vi "play-raster-scan.vi"() -> ()   [LabVIEW 2017]
uses:
  raster-scan-params.ctl
  controls/PI-params.ctl
  controls/boolean_info.ctl
  controls/raster_input_meta_data.ctl
  <vilib>/userdefined/High Color/nirio_resource_hc.ctl
  controls/rasterMetaData.ctl
  <vilib>/Utility/file.llb/Read Delimited Spreadsheet (DBL).vi
  <vilib>/FPGAPlugInAG/cRIO-9082/niLvFpga_Open_cRIO-9082.vi
  <vilib>/rvi/interface/common/dynamic/niFpgaDynamicAddResources.vi
  <vilib>/FPGAPlugInAG/Dynamic/niLvFpga_Reset_Dynamic.vi
  <vilib>/rvi/interface/common/niFpgaWaitOnOcc.vi
  <vilib>/Utility/error.llb/Error Cluster From Error Code.vi
  <vilib>/rvi/errors/niLvFpgaAdjustHostInterfaceError.vi
  <vilib>/FPGAPlugInAG/Dynamic/niLvFpga_Run_Dynamic.vi
  <vilib>/FPGAPlugInAG/Dynamic/niLvFpga_Close_Dynamic.vi
  <userlib>/_matio/level5/Public/Write/Append Data Element.llb/Append Data Element (Anything).vi
  <vilib>/rvi/interface/nirviOpenFPGA/nirviOpenFPGA.xnode
  FPGA Bitfiles/afmimagingcontro_FPGATargetSPARTA_raster-scanning_DXF4O8EAjZ4.lvbitx
  <vilib>/rvi/interface/nirviMethod/nirviMethod.xnode
  <vilib>/rvi/interface/nirviReadWriteControl/nirviReadWriteControl.xnode
  <vilib>/rvi/interface/nirviCloseFPGA/nirviCloseFPGA.xnode
  <vilib>/FPGAPlugInAG/Dynamic/niLvFpga_ConfigureFifo_Dynamic.vi
  <vilib>/rvi/errors/niLvFpgaMergeErrorWithErrorCode.vi
  <vilib>/rvi/interface/Simulation/niFpgaSimulationCallBeginRW.vi
  <vilib>/FPGAPlugInAG/Dynamic/niLvFpga_ReadFifo_Dynamic.vi
  NiFpgaLv.dll
  <userlib>/_matio/level5.lvlib
  <vilib>/FPGAPlugInAG/Dynamic/niLvFpga_WriteFifo_Dynamic.vi
panel:
  in  "detrend":bool=TRUE
  out "control":dbl[](graph)
  out "error":dbl[](graph)
  out "InputMetaData":T1
  out "output-meta-data-path":path
  in  "Tab Control":enum32{"Page 1", "Debug"}(tab)
  in  "data-root":path=path "C:/Users/arnold/Documents/labview/afm_imaging/data/raster/5microns"
  in  "number-of-pixels":i32=512
  out "points_per_line":i32=250000
  out "total_num_points":i32
  in  "raise-constant (init)":sgl
  in  "raise-constant":sgl
  in  "trigger-0":bool
  in  "STOP":bool
  in  "xy-init":fxp<+/-,16,5>[](array[numeric])=[0.0, 0.0]
  in  "Ki-xy":dbl=0.01 format="%#_13g"
  out "ADC-zaxis":sgl
  out "DAC-zaxis":sgl
  in  "xy-bound":sgl=7.0
  out "output-data-path":path
  in  "input-data-file-name":string="raster_scan_5mic_1Hz.csv"
  in  "note-blob":string
  in  "overwrite":bool
  in  "raster-scan-params":T2={"TsTicks"=1600, "Stop"=TRUE, "TOL"=0.3, "ramp-rate"=-5e-05, "z-u-max"=5.0, "PI-params"={"Ki"=0.01, "setpoint"=0.0}, "Num"=[1.0, 0.0, 0.0, 0.0, 0.0, 0.0, 0.0, 0.0, 0.0], "TF Order"=1, "Den"=[1.0, 0.0, 0.0, 0.0, 0.0, 0.0, 0.0, 0.0, 0.0]} {"ramp-rate" format="%#_5g"; "TOL" format="%#_13g"}
  in  "do-Dz":bool
  in  "do_xy_CL":bool
  out "boolean errors":T4
  in  "Z-settle-N":i16=10000
  out "Actual Depth":u32
  out "Elements Remaining":u32
  out "size(s)":i32
  out "y iter":i32
  out "nsamps 2":i32
  out "Empty Elements Remaining":u32
  out "(int) y*floor(x/y)":u64
  out "elements left 2":i32=1
  out "x >= y?":bool
  out "writing stopped":bool
  out "size(s) 2":i32
  out "case-selector-feedback":i16
  out "e(0) (threshhold init)":fxp<+/-,16,5>
  out "total-time":dbl
  out "x+1":i32
  out "que timed out?":bool
  out "Error signal (previous line) 2":dbl[](graph)
  out "Waveform Graph":dbl[](graph)
  out "base y_ref (ramp)":dbl[](graph)
  out "base x_ref(triangle wave)":dbl[](graph)
  out "Intensity Graph":dbl[][](graph)
  out "Error signal (previous line)":dbl[](graph)
  # "x-axis"
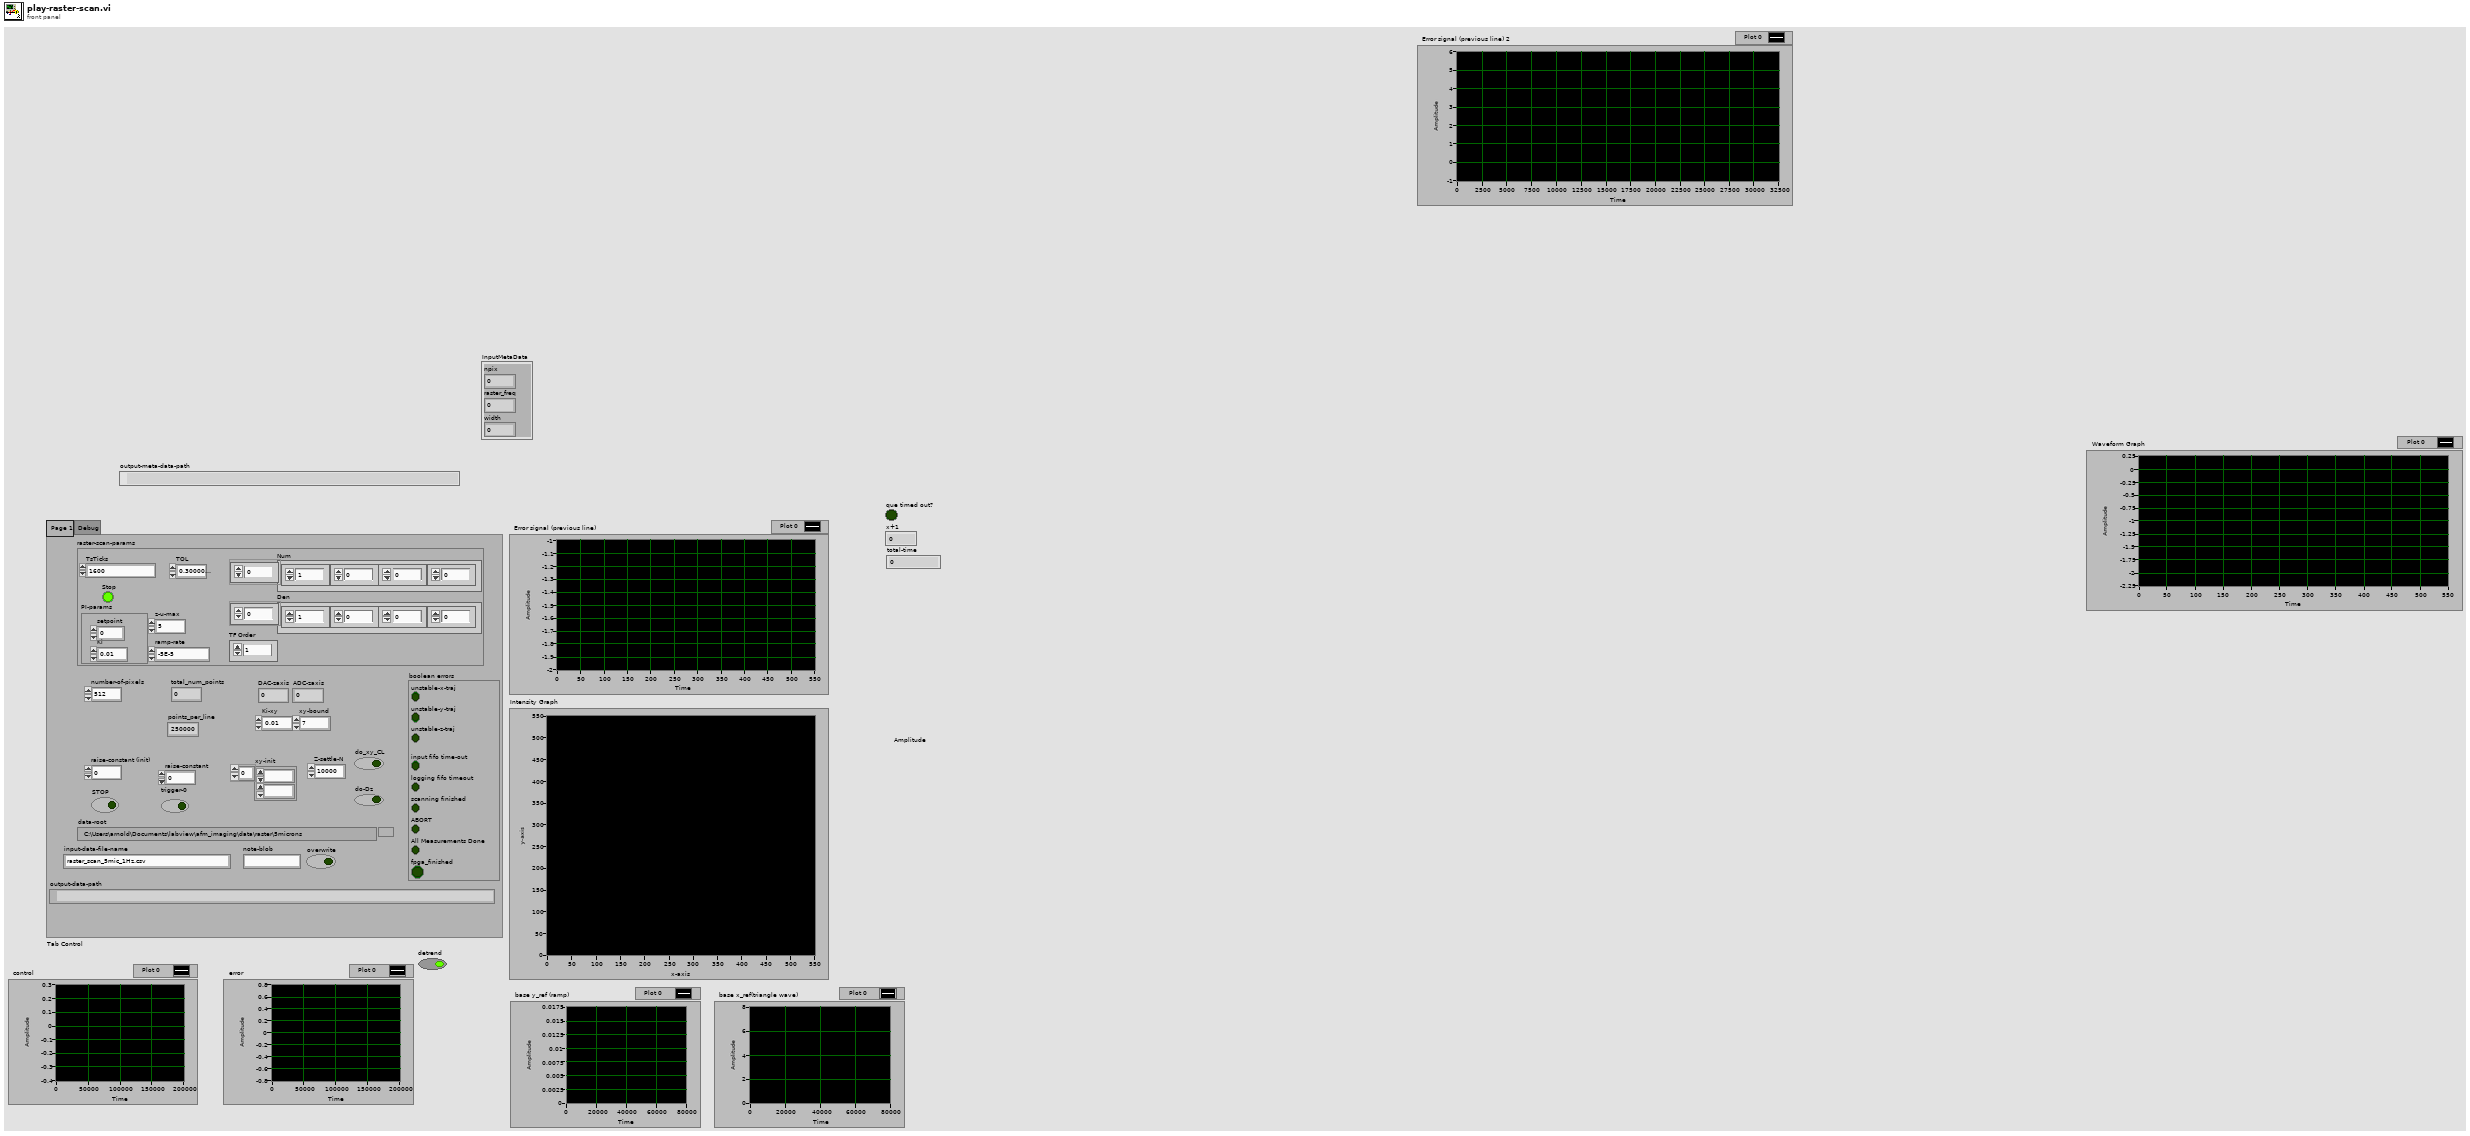
[diagram p1: front panel]
types:
  T1 = typedef "raster_input_meta_data.ctl" = cluster{"npix":dbl, "raster_freq":dbl, "width":dbl}
  T2 = typedef "raster-scan-params.ctl" = cluster{"TsTicks":u32, "Stop":bool, "TOL":sgl, "ramp-rate":sgl, "z-u-max":sgl, "PI-params":T3, "Num":sgl[], "TF Order":i32, "Den":sgl[]}
  T3 = typedef "PI-params.ctl" = cluster{"Ki":sgl, "setpoint":sgl}
  T4 = typedef "boolean_info.ctl" = cluster{"unstable-z-traj":bool, "input fifo time-out":bool, "logging fifo timeout":bool, "scanning finished":bool, "unstable-x-traj":bool, "unstable-y-traj":bool, "ABORT":bool, "All Measurements Done":bool, "fpga_finished":bool}
  T5 = typedef "nirio_resource_hc.ctl" = tag
  T6 = enum16{"open", "replace", "create", "open or create", "replace or create", "replace or create with confirmation"}
  T7 = cluster{"unstable-z-traj":bool, "input fifo time-out":bool, "logging fifo timeout":bool, "scanning finished":bool, "unstable-x-traj":bool, "unstable-y-traj":bool, "ABORT":bool, "All Measurements Done":bool, "fpga_finished":bool}
  T8 = typedef "rasterMetaData.ctl" = cluster{"raster-scan-params":T2, "xy-bound":sgl, "DAC-zaxis":sgl, "ADC-zaxis":sgl, "Ki-xy":dbl, "total_num_points":i32, "points_per_line":i32, "number-of-lines":i32, "number-of-pixels":i32, "raster_meta_in":T1}
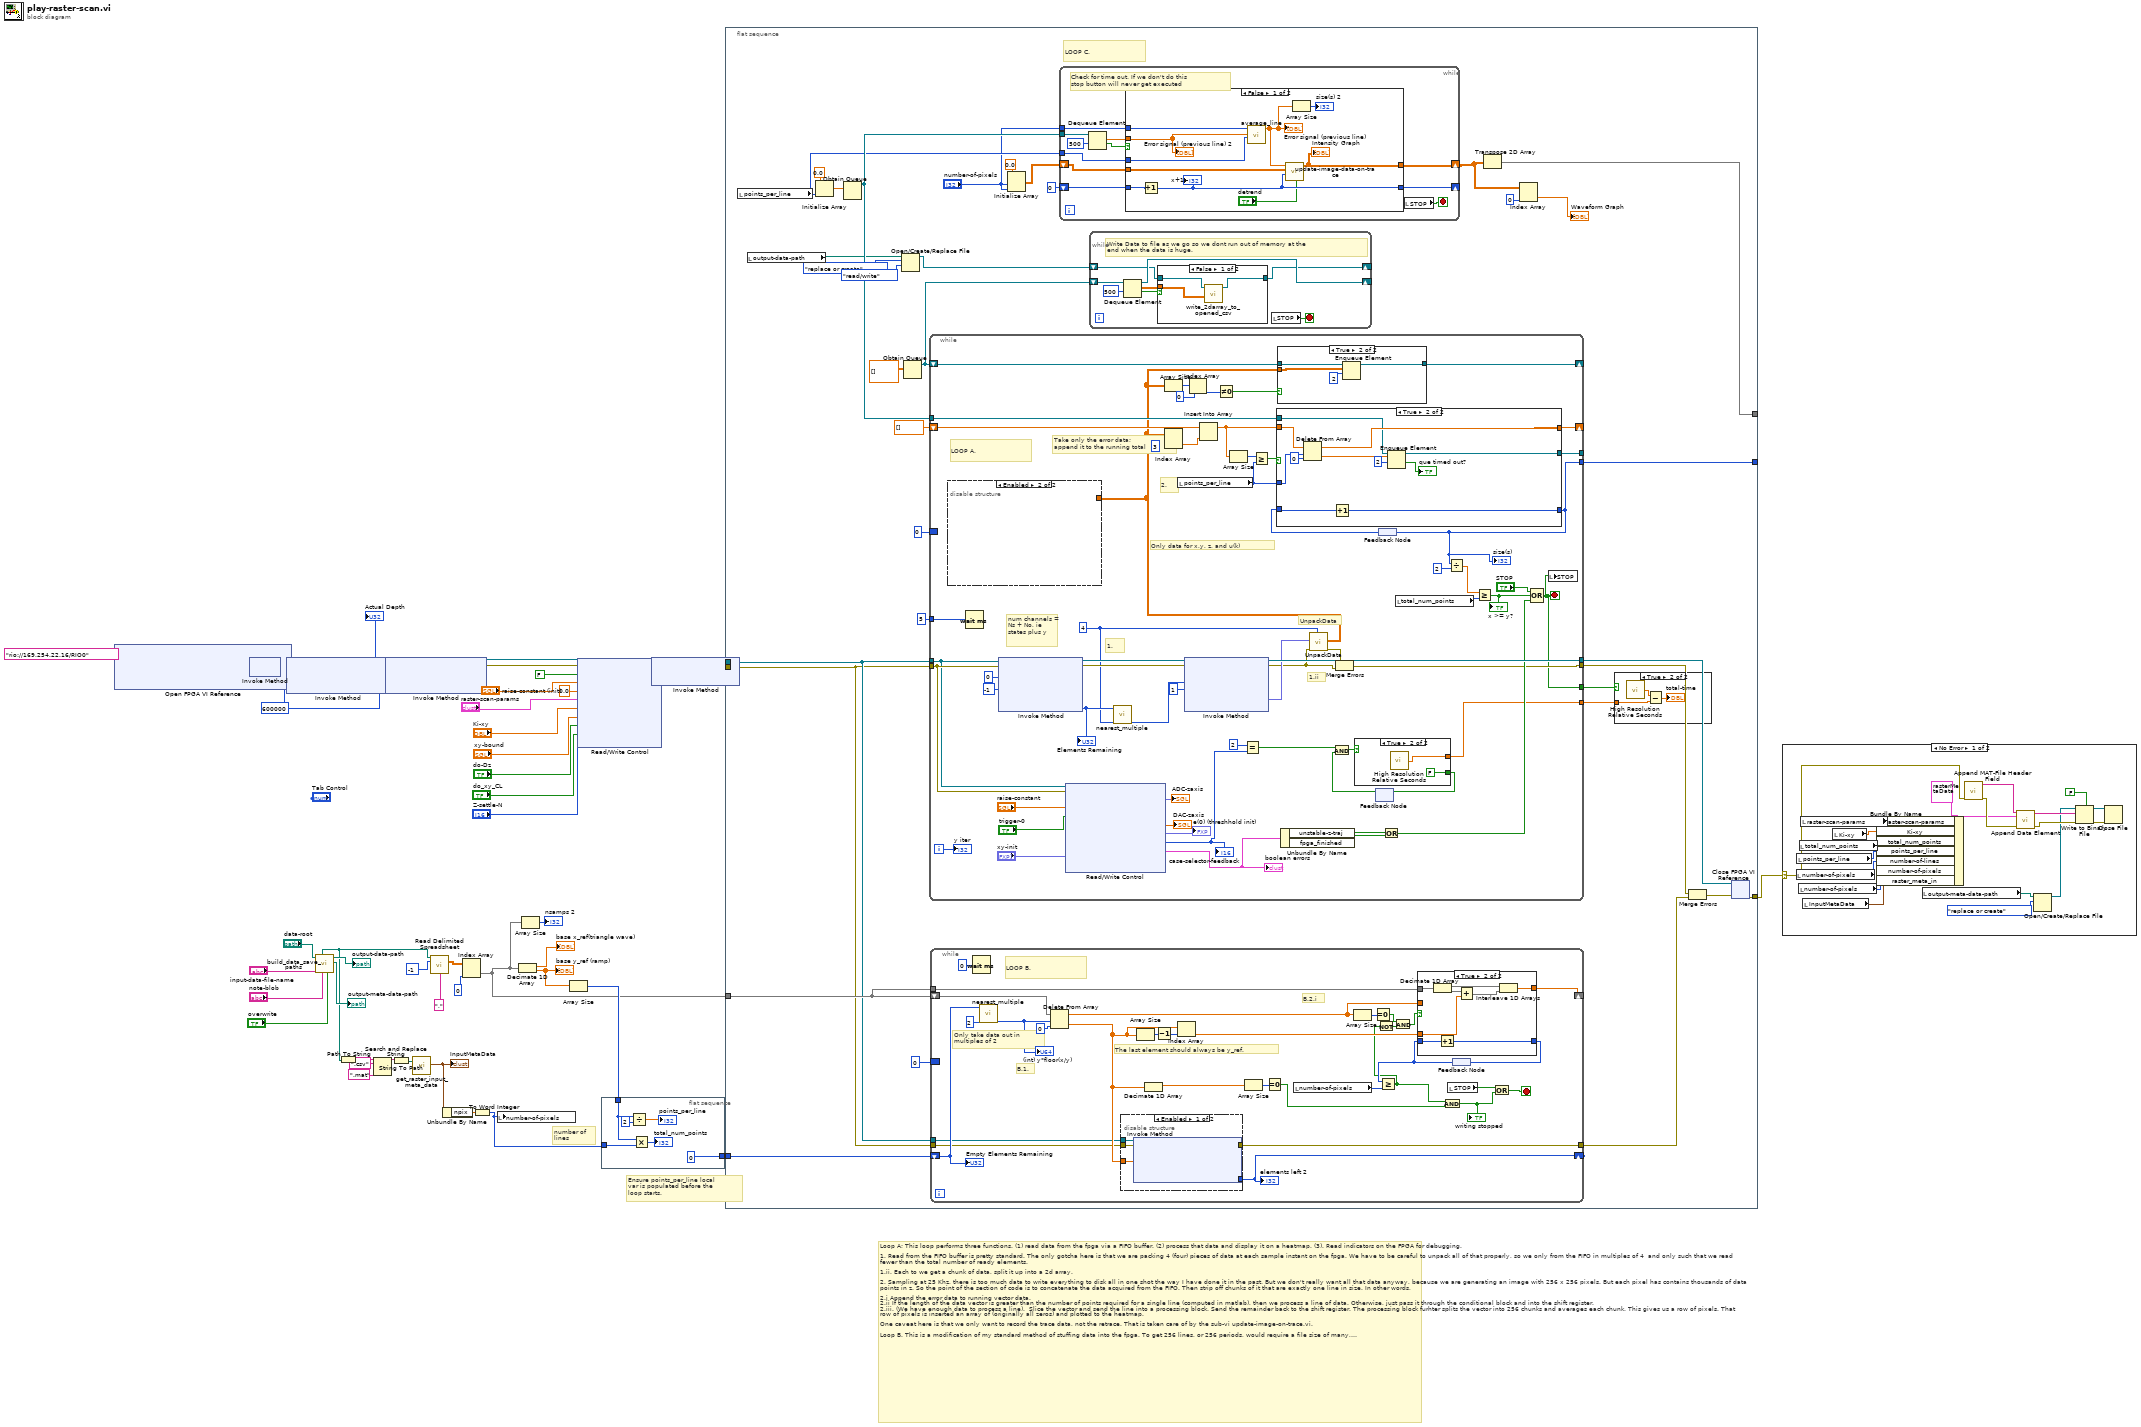
[diagram p0: block diagram]
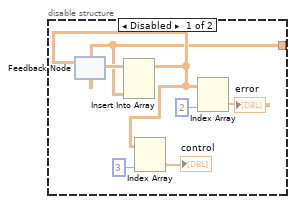
[diagram p6: hidden frame]
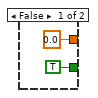
[diagram p8: hidden frame]
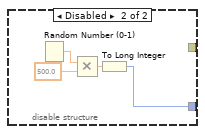
[diagram p11: hidden frame]
diagram:
  w48 = 600000
  # "number of \nlines"
  # "Loop A; This loop performs three functions. (1) read data from the fpga via a FIFO buffer. (2) process that data and display it on a heatmap. (3). Read indicators on the FPGA for debugging.\n\n1. Read from the FIFO buffer is pretty standard. The only gotcha here is that we are packing 4 (four) pieces of data at each sample instant on the fpga. We have to be careful to unpack all of that properly, so we only from the FIFO in multiples of 4  and only such that we read fewer than the total number of ready elements. \n\n1.ii. Each to we get a chunk of data, split it up into a 2d array. \n\n2. Sampling at 25 Khz, there is too much data to write everything to disk all in one shot the way I have done it in the past. But we don't really want all that data anyway, because we are generating an image with 256 x 256 pixels. But each pixel has contains thousands of data points in z. So the point of the section of code is to concatenate the data acquired from the FIFO. Then strip off chunks of it that are exactly one line in size. In other words,\n\n2.i Append the error data to running vector data.\n2.ii If the length of the data vector is greater than the number of points required for a single line (computed in matlab), then we process a line of data. Otherwise, just pass it through the conditional block and into the shift register. \n2.iii. (We have enough data to process a line).  Slice the vector and send the line into a processing block. Send the remainder back to the shift register. The processing block furhter splits the vector into 256 chunks and averages each chunk. This gives us a row of pixels. That row of pixels is inserted an array of (originally all zeros) and plotted to the heatmap.\n\nOne caveat here is that we only want to record the trace data, not the retrace. That is taken care of by the sub-vi update-image-on-trace.vi.\n\nLoop B. This is a modification of my standard method of stuffing data into the fpga. To get 256 lines, or 256 periods, would require a file size of many, many gigibtyes. SO the point here is to only use a single period of the triangle wave and corresponding ramp signal. Everytime we exauhst that data, re-cycle the same data and keep pumping it back in. The one tricky part here is that we have to be careful to shift the original ramp data up by the appropriate amount. We also have to take special care because of how the data is packed from matlab. [x(1), y(1), x(2), y(2)...].\n\nThe first iteration of the loop, we don't push any data in. All we do is get the number of empty elements.\n\nB.1 Each iteration, strip off ' empty elements ' elements from the array and send them to FIFO. \nB.2.i Is the remaining array empty?\nB.2.ii Grab the very last element. We need this"
  # "Ensure points_per_line local\nvar is populated before the\nloop starts."
  n1 = xnode "Open FPGA VI Reference"("resource name"=T5 "rio://169.254.22.16/RIO0") -> ("FPGA VI Reference Out"=w47:refnum<k20>, "error out"=w46:errorcluster)  [unwired: 1 in]
  n2 = xnode "Invoke Method"("FPGA VI Reference In"=w47, "error in"=w46) -> ("FPGA VI Reference Out"=w42:refnum<k20>, "error out"=w41:errorcluster)
  n3 = xnode "Invoke Method"("FPGA VI Reference In"=w42, "error in"=w41, "Requested Depth"=w48) -> ("FPGA VI Reference Out"=w43:refnum<k20>, "error out"=w44:errorcluster, "Actual Depth"=→"Actual Depth":u32)
  n4 = call "build_data_save_paths.vi"("overwrite"="overwrite", "note-blob"="note-blob", "base-file-name"="input-data-file-name", "data-root"="data-root") -> ("output-meta-data-path"=→"output-meta-data-path":path, "output-data-path"=→"output-data-path":path, "input-data-path"=w9:path)  [unwired: 3 in, 2 out]
  n5 = Path To String(path=w9) -> (string=w8:string)
  n6 = Search and Replace String(input string=w8, search string=".csv", replace string=".mat" ("replace string (\"\")")) -> (result string=w5:string)  [unwired: 5 in, 3 out]
  n7 = xnode "Invoke Method"("FPGA VI Reference In"=w43, "error in"=w44, "Requested Depth"=w48) -> ("FPGA VI Reference Out"=w50:refnum<k20>, "error out"=w49:errorcluster)  [unwired: 1 out]
  n8 = String To Path(string=w5) -> (path=w4:path)
  n9 = call "get_raster_input_meta_data.vi"("Path"=w4) -> ("cluster"=w3:T1)  [unwired: 10 in]
  "InputMetaData" <- w3
  n10 = call-poly <vilib>:"Read Delimited Spreadsheet.vi"("file path (dialog if empty)"=w9, "number of rows (all:-1)"=-1, "delimiter (\\t)"=",") -> ("all rows"=w28:dbl[][])  [unwired: 7 in, 5 out]
  n11 = Unbundle By Name(w3) -> ("npix"=w2:dbl)
  n12 = Index Array(array=w28, index (col)=0 ("dimension size")) -> (element=w27:dbl[])  [unwired: 1 in]
  n13 = To Word Integer(number=w2) -> (16bit integer=w1:i16)
  n14 = local write "number-of-pixels"(w1) -> ()
  n15 = Decimate 1D Array(w27) -> (→"base x_ref(triangle wave)":dbl[], w34:dbl[])
  "base y_ref (ramp)" <- w34
  n16 = Array Size(array=w27) -> (size(s)=→"nsamps 2":i32)
  n17 = Array Size(array=w34) -> (size(s)=w32:i32)
  n18 = xnode "Read/Write Control"("FPGA VI Reference In"=w50, "error in"=w49, "trigger-0"=FALSE ("constant 2 lower"), "raise-constant"="raise-constant (init)", "u(0)"=sgl 0.0, "raster-scan-params"="raster-scan-params", "Ki-xy"="Ki-xy", "xy-bound"="xy-bound", "do-Dz"="do-Dz", "do_xy_CL"="do_xy_CL", "Z-settle-N"="Z-settle-N") -> ("FPGA VI Reference Out"=w24:refnum<k20>, "error out"=w23:errorcluster)
  n19 = flat-sequence {
    tunnel: [0] -> w33
    tunnel: w32 -> [w52]
    tunnel: w1 -> [w55]
    frame #0 {
      n20 = Divide(x=w52, y=2) -> (x/y=→"points_per_line":dbl)
      n21 = Multiply(x=w52, y=w55) -> (x*y=→"total_num_points":i32)
    }
  }
  n22 = xnode "Invoke Method"("FPGA VI Reference In"=w24, "error in"=w23) -> ("FPGA VI Reference Out"=w21:refnum<k20>, "error out"=w22:errorcluster)  [unwired: 1 in]
  n23 = flat-sequence {
    tunnel: [w66] -> _
    tunnel: w21 -> [w75]
    tunnel: w22 -> [w74]
    tunnel: w33 -> [w87]
    tunnel: w27 -> [w76]
    tunnel: [w60] -> _
    tunnel: [w57] -> w13
    frame #0 {
      # "LOOP C."
      n24 = local read "points_per_line"() -> (w72:i32)
      n25 = local read "output-data-path"() -> (w59:path)
      n26 = Initialize Array(0.0 ("element"), w72) -> (w81:dbl[])
      n27 = Obtain Queue(element data type=w81) -> (queue out=w78:refnum<queue>)  [unwired: 4 in, 2 out]
      n28 = Open/Create/Replace File(file path (use dialog)=w59, operation (0:open)=T6."replace or create", access (0:read/write)=enum16{"read/write", "read-only", "write-only"}."read/write") -> (refnum out=w61:refnum<file>)  [unwired: 3 in, 2 out]
      n29 = Obtain Queue(element data type=dbl[][] []) -> (queue out=w64:refnum<queue>)  [unwired: 4 in, 2 out]
      n30 = while {
        tunnel: 5 -> [w187]
        tunnel: w75 -> [w178]
        tunnel: w74 -> [w179]
        tunnel: [w158] -> w69
        tunnel: [w181] -> w70
        shift-right: [w170] -> _
        shift-left: dbl[] [] -> [w168]
        border: 0 ("disabled index (col)") -> [_]
        tunnel: w78 -> [w149]
        tunnel: [w148] -> _
        tunnel: [w146] -> w68
        tunnel: [w139] -> w67
        shift-right: [w133] -> _
        shift-left: w64 -> [w132]
        tunnel: [w131] -> w60
        i -> [w177]
        stop <- w146 stop-if-true
        w155 = u32 4 ("y")
        # "2."
        # "1.ii"
        # "1."
        # "LOOP A."
        # "Take only the error data;\nappend it to the running total"
        # "num channels = Ns + No, ie states plus y"
        # "Only data for x,y, z, and u(k)"
        # "UnpackData"
        n31 = Wait (ms)(milliseconds to wait=w187) -> ()  [unwired: 1 out]
        n32 = xnode "Invoke Method"("FPGA VI Reference In"=w178, "error in"=w179, "Number of Elements"=0 ("Timeout (ms)"), "Timeout (ms)"=-1) -> ("FPGA VI Reference Out"=w183:refnum<k20>, "error out"=w184:errorcluster, "Elements Remaining"=w156:u32)  [unwired: 1 out]
        "Elements Remaining" <- w156
        n33 = xnode "Read/Write Control"("FPGA VI Reference In"=w178, "error in"=w179, "raise-constant"="raise-constant", "trigger-0"="trigger-0", "xy-init"="xy-init") -> ("ADC-zaxis"=→"ADC-zaxis":fxp<+/-,24,5>, "DAC-zaxis"=→"DAC-zaxis":sgl, "e(0) (threshhold init)"=→"e(0) (threshhold init)":fxp<+/-,16,5>, "current-case"=w145:i16, "boolean errors"=w130:T7)  [unwired: 1 in, 2 out]
        "case-selector-feedback" <- w145
        "boolean errors" <- w130
        n34 = call "nearest_multiple.vi"("numChan"=w155, "N"=w156) -> ("(int) y*floor(x/y)"=w154:u64)  [unwired: 9 in]
        n35 = local read "points_per_line"() -> (w157:i32)
        n36 = xnode "Invoke Method"("FPGA VI Reference In"=w183, "error in"=w184, "Number of Elements"=w154, "Timeout (ms)"=1) -> ("FPGA VI Reference Out"=w181:refnum<k20>, "error out"=w160:errorcluster, "Data"=w180:fxp<+/-,16,5>[])  [unwired: 1 out]
        n37 = Equal?(x=i16 2, y=w145) -> (x = y?=w143:bool)
        n38 = Unbundle By Name(w130) -> ("unstable-z-traj"=w151:bool, "fpga_finished"=w150:bool)
        n39 = call "UnpackData.vi"("NumChannels"=w155, "error In"=w160, "1D Data In"=w180) -> ("error Out"=w159:errorcluster, "2D Data Out"=w129:dbl[][])  [unwired: 7 in]
        n40 = disable-structure shown="Enabled" {
          disable-tunnel: w129 -> [w188 _]
          frame Disabled {
            n41 = feedback #1(w188) -> (w194:dbl[][])
            n42 = Insert Into Array(array=w194, new element=w188) -> (w189:dbl[][])  [unwired: 2 in]
            n43 = feedback-in #1(w189) -> ()
            n44 = Index Array(array=w189, index (col)=3 ("disabled index (col)")) -> (element=→"control":dbl[])  [unwired: 1 in]
            n45 = Index Array(array=w189, index (col)=2 ("disabled index (col)")) -> (element=→"error":dbl[])  [unwired: 1 in]
          }
          frame Enabled {
          }
        }
        n46 = Array Size(array=w129) -> (size(s)=w137:i32[])
        n47 = Index Array(array=w129, index (col)=3 ("disabled index (col)")) -> (element=w167:dbl[])  [unwired: 1 in]
        n48 = Index Array(array=w137, index=0) -> (element=w135:i32)
        n49 = Insert Into Array(array=w168, new element=w167) -> (w138:dbl[])  [unwired: 1 in]
        n50 = Not Equal To 0?(x=w135) -> (x != 0?=w134:bool)
        n51 = Array Size(array=w138) -> (size(s)=w169:i32)
        n52 = Greater Or Equal?(x=w169, y=w157) -> (x >= y?=w166:bool)
        n53 = case shown="True" w134 {
          tunnel: w132 -> [w195 w199]
          tunnel: w129 -> [_ w197]
          tunnel: [w195 w196] -> w133
          frame False {
          }
          frame True {
            n54 = Enqueue Element(queue=w199, element=w197, timeout in ms (-1)=2) -> (queue out=w196:refnum<queue>)  [unwired: 1 in, 2 out]
          }
        }
        n55 = Merge Errors(w159, w160) -> (w158:errorcluster)
        n56 = feedback #2() -> (w141:bool)  [unwired: 1 in]
        n57 = And(x=w143, y=w141) -> (x .and. y?=w144:bool)
        n58 = case shown="True" w144 {
          tunnel: [TRUE FALSE] -> w142
          tunnel: [0.0 ("relative seconds") w202] -> w139
          frame False {
          }
          frame True {
            n59 = call <vilib>:"High Resolution Relative Seconds.vi"() -> ("relative seconds"=w202:dbl)
          }
        }
        n60 = feedback-in #2(w142) -> ()
        n61 = feedback #3() -> (w165:i32)
        n62 = case shown="True" w166 {
          tunnel: [w206 w215] -> w170
          tunnel: w138 -> [w206 w217]
          tunnel: w165 -> [w205 w214]
          tunnel: [w205 w213] -> w131
          tunnel: w157 -> [_ w212]
          tunnel: w149 -> [w204 w210]
          tunnel: [w204 w209] -> w148
          frame False {
          }
          frame True {
            n63 = Delete From Array(array=w217, length=w212, index=0) -> (deleted portion=w211:dbl[], array with subset deleted=w215:dbl[])
            n64 = Increment(x=w214) -> (x+1=w213:i32)
            n65 = Enqueue Element(queue=w210, element=w211, timeout in ms (-1)=2) -> (queue out=w209:refnum<queue>, timed out?=→"que timed out?":bool)  [unwired: 1 in, 1 out]
          }
        }
        "size(s)" <- w131
        n66 = feedback-in #3(w131) -> ()
        n67 = Or(x=w151, y=w150) -> (x .or. y?=w161:bool)
        n68 = local read "total_num_points"() -> (w164:i32)
        n69 = Divide(x=w131, y=2) -> (x/y=w153:dbl)
        n70 = Greater Or Equal?(x=w153, y=w164) -> (x >= y?=w162:bool)
        "x >= y?" <- w162
        n71 = Compound Arithmetic op=OR("STOP", w162, w161) -> (w146:bool)
        n72 = local write "STOP"(w146) -> ()
        "y iter" <- w177
      }
      n73 = while {
        shift-right: [w247] -> _
        shift-left: w87 -> [w242]
        shift-right: [w235] -> _
        shift-left: w76 -> [w248]
        tunnel: w76 -> [w233]
        tunnel: [w239] -> w88
        tunnel: w75 -> [w231]
        tunnel: w74 -> [w230]
        border: 0 ("Timeout (ms)") -> [_]
        stop <- w243 stop-if-true
        # "B.2.i"
        # "B.1."
        # "LOOP B."
        # "Only take data out in \nmultiples of 2"
        # "The last element should always be y_ref."
        n74 = Wait (ms)(milliseconds to wait=0) -> ()  [unwired: 1 out]
        n75 = call "nearest_multiple.vi"("numChan"=u32 2 ("Empty Elements Remaining"), "N"=w242) -> ("(int) y*floor(x/y)"=w241:u64)  [unwired: 9 in]
        "(int) y*floor(x/y)" <- w241
        n76 = Delete From Array(array=w248, length=w241, index=0) -> (deleted portion=w236:dbl[], array with subset deleted=w234:dbl[])
        n77 = disable-structure shown="Enabled" {
          disable-tunnel: [w263 w264] -> w247
          disable-tunnel: w236 -> [w262 _]
          disable-tunnel: [w261 _] -> w239
          disable-tunnel: w231 -> [w260 _]
          disable-tunnel: w230 -> [w259 _]
          frame Enabled {
            n78 = xnode "Invoke Method"("FPGA VI Reference In"=w260, "error in"=w259, "Data"=w262) -> ("error out"=w261:errorcluster, "Empty Elements Remaining"=w263:u32)  [unwired: 1 in, 1 out]
          }
          frame Disabled {
            n79 = Random Number (0-1)() -> (number: 0 to 1=w267:dbl)
            n80 = Multiply(x=w267, y=500.0) -> (x*y=w265:dbl)
            n81 = To Long Integer(number=w265) -> (32bit integer=w264:i32)
          }
        }
        "elements left 2" <- w247
        n82 = Array Size(array=w236) -> (size(s)=w237:i32)
        n83 = Decimate 1D Array(w236) -> (w222:dbl[])  [unwired: 1 out]
        n84 = Decrement(x=w237) -> (x-1=w238:i32)
        n85 = Index Array(array=w236, index=w238) -> (element=w232:dbl)
        n86 = Array Size(array=w222) -> (size(s)=w224:i32)
        n87 = Equal To 0?(x=w224) -> (x = 0?=w223:bool)
        n88 = local read "number-of-pixels"() -> (w228:i32)
        n89 = Array Size(array=w234) -> (size(s)=w245:i32)
        n90 = Equal To 0?(x=w245) -> (x = 0?=w221:bool)
        n91 = local read "STOP"() -> (w244:bool)
        n92 = feedback #4() -> (w226:i32)
        n93 = Greater Or Equal?(x=w226, y=w228) -> (x >= y?=w219:bool)
        n94 = Not(x=w219) -> (.not. x?=w220:bool)
        n95 = And(x=w221, y=w220) -> (x .and. y?=w218:bool)
        n96 = case shown="True" w218 {
          tunnel: [w250 w253] -> w235
          tunnel: w234 -> [w250 _]
          tunnel: w233 -> [_ w258]
          tunnel: w232 -> [_ w256]
          tunnel: [w249 w252] -> w227
          tunnel: w226 -> [w249 w251]
          frame False {
          }
          frame True {
            n97 = Decimate 1D Array(w258) -> (w255:dbl[], w257:dbl[])
            n98 = Increment(x=w251) -> (x+1=w252:i32)
            n99 = Add(x=w257, y=w256) -> (x+y=w254:dbl[])
            n100 = Interleave 1D Arrays(w255, w254) -> (w253:dbl[])
          }
        }
        n101 = And(x=w219, y=w223) -> (x .and. y?=w225:bool)
        "writing stopped" <- w225
        n102 = feedback-in #4(w227) -> ()
        n103 = Or(x=w244, y=w225) -> (x .or. y?=w243:bool)
        "Empty Elements Remaining" <- w242
      }
      n104 = Initialize Array(0.0 ("element"), "number-of-pixels", "number-of-pixels") -> (w80:dbl[][])
      n105 = while {
        shift-right: [w116] -> w77
        shift-left: w80 -> [w115]
        shift-right: [w113] -> _
        shift-left: 0 ("disabled index (col)") -> [w114]
        tunnel: w72 -> [w112]
        tunnel: w78 -> [w111]
        tunnel: "number-of-pixels" -> [w106]
        stop <- w109 stop-if-true
        # "Check for time out. If we don't do this\nstop button will never get executed"
        n106 = Dequeue Element(queue=w111, timeout in ms (-1)=500) -> (element=w110:dbl[], timed out?=w107:bool)  [unwired: 1 in, 2 out]
        n107 = case shown="False" w107 {
          tunnel: [w126 w127] -> w116
          tunnel: w115 -> [w125 w127]
          tunnel: w114 -> [w124 w128]
          tunnel: [w123 w128] -> w113
          tunnel: w112 -> [w122 _]
          tunnel: w110 -> [w121 _]
          tunnel: w106 -> [w118 _]
          frame False {
            n108 = Increment(x=w124) -> (x+1=w123:i32)
            "x+1" <- w123
            n109 = call "average_line.vi"("data-pts-per-line"=w122, "raw-data-row"=w121, "number-of-pixels"=w118) -> ("avg-data-row"=w120:dbl[])  [unwired: 8 in]
            "Error signal (previous line)" <- w120
            n110 = call "update-image-data-on-trace.vi"("detrend"="detrend", "iterator"=w123, "master-image-data-n"=w125, "avg-data-row"=w120) -> ("master-image-data-out"=w126:dbl[][])  [unwired: 7 in]
            "Intensity Graph" <- w126
            n111 = Array Size(array=w120) -> (size(s)=→"size(s) 2":i32)
            "Error signal (previous line) 2" <- w121
          }
          frame True {
          }
        }
        n112 = local read "STOP"() -> (w109:bool)
      }
      n113 = while {
        shift-right: [w93] -> _
        shift-left: w64 -> [w94]
        shift-right: [w91] -> _
        shift-left: w61 -> [w92]
        stop <- w96 stop-if-true
        # "Write Data to file as we go so we dont run out of memory at the \nend when the data is huge."
        n114 = Dequeue Element(queue=w94, timeout in ms (-1)=500) -> (queue out=w93:refnum<queue>, element=w95:dbl[][], timed out?=w97:bool)  [unwired: 1 in, 1 out]
        n115 = case shown="False" w97 {
          tunnel: w95 -> [w99 _]
          tunnel: w92 -> [w101 w102]
          tunnel: [w100 w102] -> w91
          frame False {
            n116 = call "write_2darray_to_opened_csv.vi"("Data_in"=w99, "file_ref_in"=w101) -> ("file_ref_out"=w100:refnum<file>)  [unwired: 9 in]
          }
          frame True {
          }
        }
        n117 = local read "STOP"() -> (w96:bool)
      }
      n118 = Transpose 2D Array(2D array=w77) -> (transposed array=w66:dbl[][])
      n119 = Index Array(array=w77, index (col)=0 ("disabled index (col)")) -> (element=→"Waveform Graph":dbl[])  [unwired: 1 in]
      n120 = case shown="True" w68 {
        tunnel: w67 -> [_ w105]
        frame False {
        }
        frame True {
          n121 = call <vilib>:"High Resolution Relative Seconds.vi"() -> ("relative seconds"=w104:dbl)
          n122 = Subtract(x=w104, y=w105) -> (x-y=→"total-time":dbl)
        }
      }
      n123 = Merge Errors(w69, w88) -> (w58:errorcluster)
      n124 = xnode "Close FPGA VI Reference"("FPGA VI Reference In"=w70, "error in"=w58) -> ("error out"=w57:errorcluster)
    }
  }
  n125 = case shown="No Error" w13 {
    selector: w13 -> [w276 _]
    frame No Error {
      n126 = local read "number-of-pixels"() -> (w270:i32)
      n127 = local read "points_per_line"() -> (w271:i32)
      n128 = local read "number-of-pixels"() -> (w269:i32)
      n129 = local read "total_num_points"() -> (w272:i32)
      n130 = local read "raster-scan-params"() -> (w274:T2)
      n131 = local read "InputMetaData"() -> (w268:T1)
      n132 = local read "Ki-xy"() -> (w273:dbl)
      n133 = Bundle By Name(cluster=T8 {"raster-scan-params"={"TsTicks"=1600, "Stop"=TRUE, "TOL"=0.3, "ramp-rate"=-5e-05, "z-u-max"=5.0, "PI-params"={"Ki"=0.01, "setpoint"=0.0}, "Num"=[1.0, 0.0, 0.0, 0.0, 0.0, 0.0, 0.0, 0.0, 0.0], "TF Order"=3, "Den"=[1.0, 0.0, 0.0, 0.0, 0.0, 0.0, 0.0, 0.0, 0.0]}, "xy-bound"=7.0, "DAC-zaxis"=0.0, "ADC-zaxis"=0.0, "Ki-xy"=0.01, "total_num_points"=0, "points_per_line"=250000, "number-of-lines"=256, "number-of-pixels"=256, "raster_meta_in"={"npix"=0.0, "raster_freq"=0.0, "width"=0.0}} ("Cluster"), "raster-scan-params"=w274, "Ki-xy"=w273, "total_num_points"=w272, "points_per_line"=w271, "number-of-lines"=w270, "number-of-pixels"=w269, "raster_meta_in"=w268) -> (w275:T8)
      n134 = local read "output-meta-data-path"() -> (w278:path)
      n135 = call <userlib>:"Append MAT-File Header Field.vi"("error"=w276) -> ("result string"=w287:string, "error out"=w281:errorcluster)  [unwired: 13 in]
      n136 = call-poly <userlib>:"Append Data Element.vi"("initial string"=w287, "data"=w275, "error in (no error)"=w281) -> ("result string"=w285:string, "error out"=w286:errorcluster)  [unwired: 11 in]
      n137 = Open/Create/Replace File(file path (use dialog)=w278, operation (0:open)=T6."replace or create") -> (refnum out=w280:refnum<file>)  [unwired: 4 in, 2 out]
      n138 = Write to Binary File(file (use dialog)=w280, data=w285, error in=w286, 5:FALSE ("prepend array or string size? (T)")) -> (refnum out=w282:refnum<file>, error out=w283:errorcluster)  [unwired: 2 in, 1 out]
      n139 = Close File(refnum=w282, error in=w283) -> ()  [unwired: 2 out]
    }
    frame Error {
    }
  }
